vi "overlay target circles.vi"(3 "Color":u32, 4 "CamConfigArray":T2, 5 "Image Dst Out":T3) -> (0 "Cluster":cluster{"X Target":sgl, dbl}, 1 "Image Out":T3, 2 "Numeric":dbl)   [LabVIEW 2013]
uses:
  <vilib>/vision/Image Controls.llb/IMAQ Image.ctl
  <vilib>/userdefined/High Color/IMAQdx.ctl
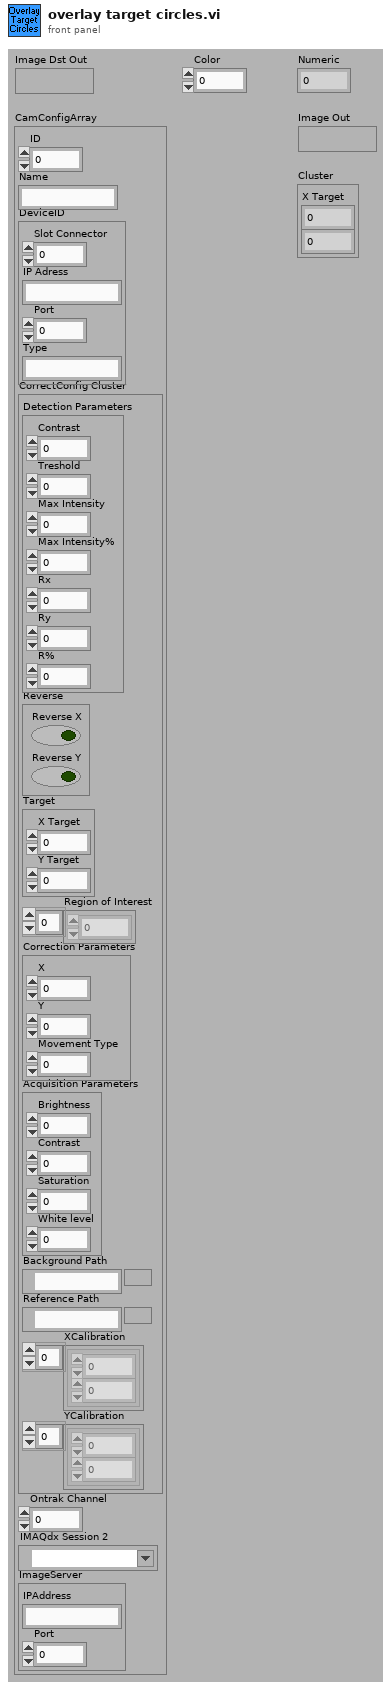
[diagram p1: front panel]
types:
  T1 = typedef "IMAQdx.ctl" = refnum<k21>
  T2 = cluster{"ID":dbl, "Name":string, "DeviceID":cluster{"Slot Connector":i32, "IP Adress":string, "Port":i32, "Type":string}, "CorrectConfig Cluster":cluster{"Detection Parameters":cluster{"Contrast":i32, "Treshold":u8, "Max Intensity":i32, "Max Intensity%":u8, "Rx":i32, "Ry":i32, "R%":sgl}, "Reverse":cluster{"Reverse X":bool, "Reverse Y":bool}, "Target":cluster{"X Target":sgl, "Y Target":sgl}, "Region of Interest":i32[], "Correction Parameters":cluster{"X":sgl, "Y":sgl, "Movement Type":u16}, "Acquisition Parameters":cluster{"Brightness":dbl, "Contrast":dbl, "Saturation":dbl, "White level":dbl}, "Background Path":path, "Reference Path":path, "XCalibration":cluster{dbl, dbl}[], "YCalibration":cluster{dbl, dbl}[]}, "Ontrak Channel":i16, "IMAQdx Session 2":T1, "ImageServer":cluster{"IPAddress":string, "Port":i32}}
  T3 = typedef "IMAQ Image.ctl" = refnum<image>
  T4 = cluster{"Left":i32, "Top":i32, "Right":i32, "Bottom":i32}
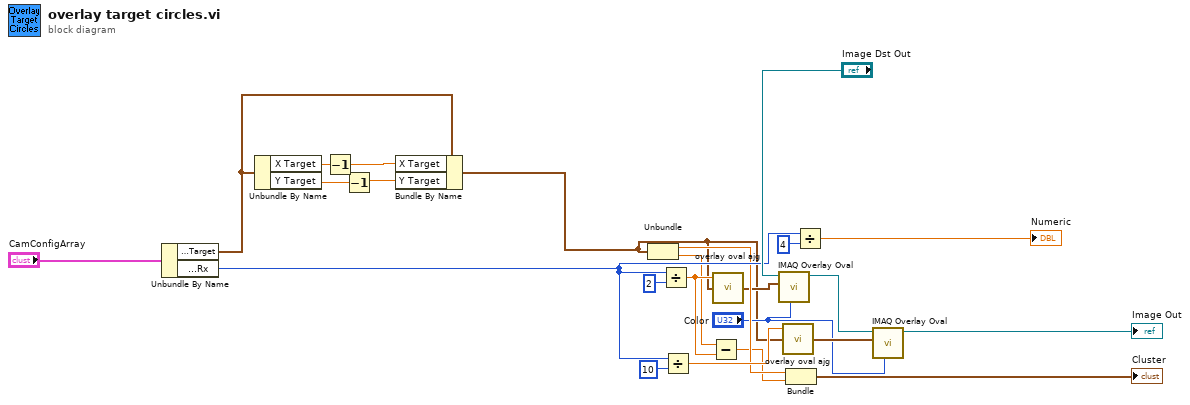
[diagram p0: block diagram]
diagram:
  n1 = Unbundle By Name("CamConfigArray") -> ("CorrectConfig Cluster.Target"=w4:cluster{"X Target":sgl, "Y Target":sgl}, "CorrectConfig Cluster.Detection Parameters.Rx"=w21:i32)
  n2 = Unbundle By Name(w4) -> ("X Target"=w6:sgl, "Y Target"=w5:sgl)
  n3 = Decrement(x=w6) -> (x-1=w3:sgl)
  n4 = Decrement(x=w5) -> (x-1=w2:sgl)
  n5 = Bundle By Name(cluster=w4, "X Target"=w3, "Y Target"=w2) -> (w1:cluster{"X Target":sgl, "Y Target":sgl})
  n6 = Unbundle(w1) -> ("X Target"=w17:sgl, "Y Target"=w15:sgl)
  n7 = Divide(x=w21, y=2 ("CorrectConfig Cluster.Detection Parameters.Rx")) -> (x/y=w23:dbl)
  n8 = Divide(x=w21, y=10 ("CorrectConfig Cluster.Detection Parameters.Rx")) -> (x/y=w22:dbl)
  n9 = Subtract(x=w15, y=w23) -> (x-y=w16:dbl)
  n10 = call "overlay oval ajg.vi"("xy coords"=w1, "Circle R"=w23) -> ("Bounding Rectangle"=w7:T4)  [unwired: 1 in]
  n11 = call "IMAQ Overlay Oval"("Color"="Color", "Bounding Rectangle"=w7, "Image"="Image Dst Out") -> ("Image Out"=w10:T3)  [unwired: 7 in, 1 out]
  n12 = call "overlay oval ajg.vi"("xy coords"=w1, "Circle R"=w22) -> ("Bounding Rectangle"=w14:T4)  [unwired: 1 in]
  n13 = Bundle("X Target"=w17, w16) -> (→"Cluster":cluster{"X Target":sgl, dbl})  [unwired: 1 in]
  n14 = Divide(x=w21, y=4 ("CorrectConfig Cluster.Detection Parameters.Rx")) -> (x/y=→"Numeric":dbl)
  n15 = call "IMAQ Overlay Oval"("Color"="Color", "Bounding Rectangle"=w14, "Image"=w10) -> ("Image Out"=→"Image Out":T3)  [unwired: 7 in, 1 out]
